vi "GetVoltageRef.vi"(8 "error in (no error)":errorcluster, 9 "lsecon":T1={"NoiseVariance"=0.001, "IEEESystem"=5, "PMULocations"=[1], "Vindex"=0, "Iindex"=3, "DynamicRef"=""}, 10 "SystemVoltagesRef":cdb[][](array[numeric])) -> (0 "error out":errorcluster, 2 "SystemVoltagesRef Out":cdb[][](array[numeric]))   [LabVIEW 2014, in "AppPlugins.lvlib" / "LSEPlugin.lvclass"]
uses:
  LSEPlugin.lvclass
  Typedefs/LSEConfig.ctl
  <vilib>/Utility/file.llb/Read From Spreadsheet File (string).vi
  Visualization/VisualizeApp_class/VisualizeAppLSE.lvclass
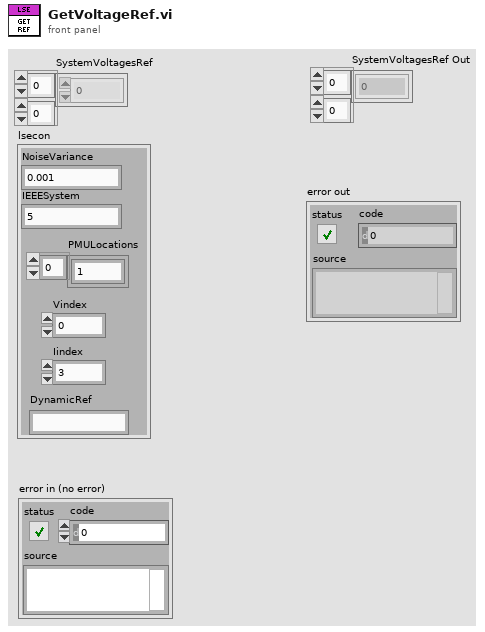
[diagram p1: front panel]
types:
  T1 = typedef "AppPlugins.lvlib/LSEPlugin.lvclass/LSEConfig.ctl" = cluster{"NoiseVariance":dbl, "IEEESystem":u32, "PMULocations":u32[], "Vindex":i32, "Iindex":i32, "DynamicRef":string}
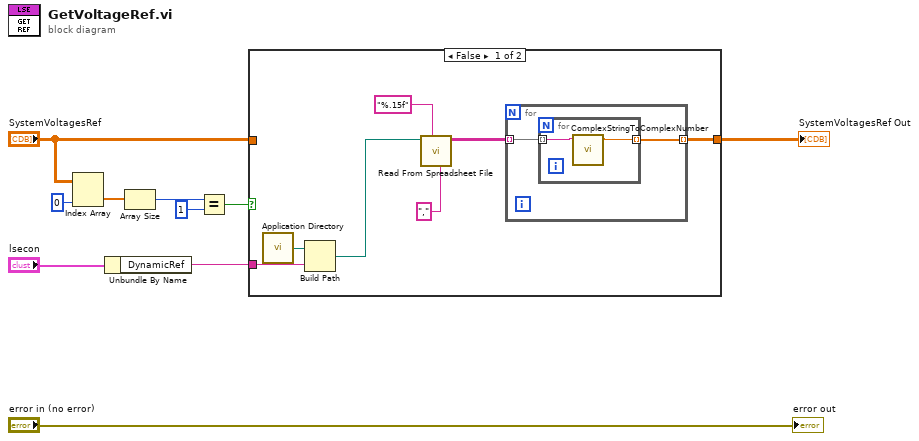
[diagram p0: block diagram]
diagram:
  n1 = Index Array(array="SystemVoltagesRef", index (col)=0 ("disabled index (col)")) -> (element=w3:cdb[])  [unwired: 1 in]
  n2 = Unbundle By Name("lsecon") -> ("DynamicRef"=w1:string)
  n3 = Array Size(array=w3) -> (size(s)=w8:i32)
  n4 = Equal?(x=w8, y=1) -> (x = y?=w6:bool)
  n5 = case shown="False" w6 {
    tunnel: [w14 w22] -> w9
    tunnel: "SystemVoltagesRef" -> [_ w22]
    tunnel: w1 -> [w12 _]
    frame False {
      n6 = call <vilib>:"Application Directory.vi"() -> ("Application Directory"=w13:path)
      n7 = Build Path(base path=w13, name or relative path=w12) -> (appended path=w11:path)
      n8 = call-poly <vilib>:"Read From Spreadsheet File.vi"("delimiter (\\t)"="," ("delimiter (\\t)"), "format (%s)"="%.15f" ("format (%.3f)"), "file path (dialog if empty)"=w11) -> ("all rows"=w15:string[][])  [unwired: 4 in, 4 out]
      n9 = for {
        tunnel: w15 -> [w19] mode=indexing
        tunnel: [w18] -> w14 mode=indexing
        n10 = for {
          tunnel: w19 -> [w21] mode=indexing
          tunnel: [w20] -> w18 mode=indexing
          n11 = call "ComplexStringToComplexNumber.vi"("String"=w21) -> ("Numeric"=w20:cdb)  [unwired: 10 in]
        }
      }
    }
    frame True {
    }
  }
  "SystemVoltagesRef Out" <- w9
  "error out" <- "error in (no error)"
